vi "Rx Streaming (Host).vi"() -> ()   [LabVIEW 2015]
doc: "This template is for the Simple NI-USRP Streaming design, a design that shows the basics of streaming data to and from an NI USRP-294x/295x device. Refer to the block diagram for more information about how to use this template."
uses:
  <vilib>/userdefined/Silver/nirio_resource_slv.ctl
  SubVIs/Start Trigger.ctl
  <vilib>/Utility/error.llb/DialogType.ctl
  <vilib>/imath/engines/lvmath/Plug In/_Char/NIMS_CH_character datatype.ctl
  <instrlib>/niUsrpRio/Time/v1/Host/Private/Get Time (Single).vi
  Supporting Files/Global Vars.vi
  <vilib>/imath/engines/lvmath2/RunTimeEngine/Managers/WorkSpace/UID Generator.vi
  <vilib>/imath/engines/lvmath2/RunTimeEngine/BuiltInFunctions/close/NIMS_close(Enums).vi
  <vilib>/imath/engines/lvmath2/RunTimeEngine/RunTimeType/NIMS_RunTimeType_From StrictType (excl LVString).vi
  <instcachedir>/0/NIMS_RunTimeType_From StrictType (excl LVString)_EB1C38A9BC5048DA9ABDA8F781E54D21.lvgen/NIMS_RunTimeType_From StrictType (excl LVString)_EB1C38A9BC5048DA9ABDA8F781E54D21_000.vi
  <vilib>/imath/engines/lvmath2/RunTimeEngine/LocalVariableDefStatement/MC_LocalVariableDefStatement_Display.vi
  <vilib>/imath/engines/lvmath2/RunTimeEngine/BuiltInFunctions/log2/NIMS_log2(1o).vi
  <instcachedir>/0/NIMS_log2(1o)_7A1FF839A5EC4375BBB20124C6B1C03A.lvgen/NIMS_log2(1o)_7A1FF839A5EC4375BBB20124C6B1C03A_001.vi
  <vilib>/imath/engines/lvmath2/RunTimeEngine/RangeToken/NIMS_Range_R2 - Float.vi
  <instcachedir>/0/NIMS_Range_R2 - Float_98052C3F8D284261A146188355820AF0.lvgen/NIMS_Range_R2 - Float_98052C3F8D284261A146188355820AF0_000.vi
  <vilib>/imath/engines/lvmath2/RunTimeEngine/CommandStatement/MC_CommandStatement_break.vi
  <vilib>/imath/engines/lvmath2/RunTimeEngine/VariableToken/NIMS_VariableToken_CondDefined.vi
  <instcachedir>/0/NIMS_VariableToken_CondDefined_FE30D0A1BFB24F098D41DEBABFE96BE1.lvgen/NIMS_VariableToken_CondDefined_FE30D0A1BFB24F098D41DEBABFE96BE1_003.vi
  <vilib>/imathl/engines/lvmath/Functions/Error Handling/Create Error.vi
  <vilib>/imath/engines/lvmath2/RunTimeEngine/BuiltInFunctions/zeros/NIMS_V=zeros(I32,I32).vi
  <vilib>/imath/engines/lvmath2/RunTimeEngine/IndexRead/NIMS V(R2).vi
  <instcachedir>/0/NIMS V(R2)_C76619605A0E4E9F8B2FA9389712AC47.lvgen/NIMS V(R2)_C76619605A0E4E9F8B2FA9389712AC47_002.vi
  <vilib>/imath/engines/lvmath2/RunTimeEngine/ErrorHandling/NIMS_Create Error From Enums.vi
  <vilib>/imath/engines/lvmath2/RunTimeEngine/BuiltInFunctions/fftshift/NIMS_fftshift(GV).vi
  <instcachedir>/0/NIMS_fftshift(GV)_BD7A7BA9CA6B470B9A9F73A6A3FEEB3E.lvgen/NIMS_fftshift(GV)_BD7A7BA9CA6B470B9A9F73A6A3FEEB3E_000.vi
  <vilib>/imath/engines/lvmath2/RunTimeEngine/BuiltInFunctions/length/NIMS_length(GV).vi
  <instcachedir>/0/NIMS_length(GV)_08A3D13377FD4E4B96F5795FBF3698FA.lvgen/NIMS_length(GV)_08A3D13377FD4E4B96F5795FBF3698FA_004.vi
  <instcachedir>/0/NIMS V(R2)_C76619605A0E4E9F8B2FA9389712AC47.lvgen/NIMS V(R2)_C76619605A0E4E9F8B2FA9389712AC47_004.vi
  <vilib>/imath/engines/lvmath2/RunTimeEngine/BuiltInFunctions/fft/NIMS_fft(GV).vi
  <instcachedir>/0/NIMS_fft(GV)_4C6467FC22F84E4BA42517A07EF978B0.lvgen/NIMS_fft(GV)_4C6467FC22F84E4BA42517A07EF978B0_001.vi
  <instcachedir>/0/NIMS_fftshift(GV)_BD7A7BA9CA6B470B9A9F73A6A3FEEB3E.lvgen/NIMS_fftshift(GV)_BD7A7BA9CA6B470B9A9F73A6A3FEEB3E_001.vi
  <vilib>/imath/engines/lvmath2/RunTimeEngine/ErrorHandling/NIMS_Error From Error Code.vi
  <vilib>/imath/engines/lvmath2/RunTimeEngine/BuiltInFunctions/mean/NIMS_CS=mean(CV,I32).vi
  <vilib>/imath/engines/lvmath2/RunTimeEngine/RangeToken/NIMS_Range.vi
  <instcachedir>/0/NIMS_Range_D919CC09935940E88F755EC1C6F49AC1.lvgen/NIMS_Range_D919CC09935940E88F755EC1C6F49AC1_000.vi
  <vilib>/imath/engines/lvmath2/RunTimeSupport/NIMS_Error if Not Equal.vi
  <instcachedir>/0/NIMS_Error if Not Equal_7F0D61CE56BF44979916ECA34C78675F.lvgen/NIMS_Error if Not Equal_7F0D61CE56BF44979916ECA34C78675F_001.vi
  <vilib>/imath/engines/lvmath2/RunTimeEngine/IndexRead/NIMS V(V).vi
  <instcachedir>/0/NIMS V(V)_298D9CB7BFEB42B8BC8D9C3C28AE8C70.lvgen/NIMS V(V)_298D9CB7BFEB42B8BC8D9C3C28AE8C70_000.vi
  <vilib>/imath/engines/lvmath2/RunTimeEngine/ArithmeticOperatorToken/NIMS_ArithmeticOperator_times.vi
  <instcachedir>/0/NIMS_ArithmeticOperator_times_DF26C4080E2A467BA28C929B8CF31953.lvgen/NIMS_ArithmeticOperator_times_DF26C4080E2A467BA28C929B8CF31953_003.vi
  <vilib>/imath/engines/lvmath2/RunTimeEngine/BuiltInFunctions/sum/NIMS_sum(GV).vi
  <instcachedir>/0/NIMS_sum(GV)_67F5EC36BC034E54A6BEC5B0673C00E5.lvgen/NIMS_sum(GV)_67F5EC36BC034E54A6BEC5B0673C00E5_001.vi
  <vilib>/imath/engines/lvmath2/RunTimeEngine/BuiltInFunctions/conjugate/NIMS_conjugate(Complex).vi
  <instcachedir>/0/NIMS_conjugate(Complex)_151E186CA54B4853A0120BB0A667D86E.lvgen/NIMS_conjugate(Complex)_151E186CA54B4853A0120BB0A667D86E_001.vi
  <vilib>/imath/engines/lvmath2/RunTimeEngine/IndexRead/NIMS V(R3).vi
  <instcachedir>/0/NIMS V(R3)_BB7B7B2F47B844E7B6C44853B6A6C035.lvgen/NIMS V(R3)_BB7B7B2F47B844E7B6C44853B6A6C035_000.vi
  <instcachedir>/0/NIMS V(R2)_C76619605A0E4E9F8B2FA9389712AC47.lvgen/NIMS V(R2)_C76619605A0E4E9F8B2FA9389712AC47_001.vi
  <instcachedir>/0/NIMS_conjugate(Complex)_151E186CA54B4853A0120BB0A667D86E.lvgen/NIMS_conjugate(Complex)_151E186CA54B4853A0120BB0A667D86E_002.vi
  <vilib>/imath/engines/lvmath2/RunTimeEngine/ArithmeticOperatorToken/NIMS_ArithmeticOperator_minus.vi
  <instcachedir>/0/NIMS_ArithmeticOperator_minus_8228ED1EA52B4CB8A68367813E4B0C9D.lvgen/NIMS_ArithmeticOperator_minus_8228ED1EA52B4CB8A68367813E4B0C9D_000.vi
  <vilib>/imath/engines/lvmath2/RunTimeEngine/IndexReplace/NIMS V(R2)=V.vi
  <instcachedir>/0/NIMS V(R2)=V_A4A1DC5DDA874862BD08E3229D1DC268.lvgen/NIMS V(R2)=V_A4A1DC5DDA874862BD08E3229D1DC268_000.vi
  <vilib>/imath/engines/lvmath2/RunTimeEngine/BuiltInFunctions/ifft/NIMS_ifft(CV).vi
  <vilib>/imath/engines/lvmath2/RunTimeEngine/BuiltInFunctions/circularshift/NIMS_circularshift(GRowV,V).vi
  <instcachedir>/0/NIMS_circularshift(GRowV,V)_5CE594553FE04FE4B0327743CF19F361.lvgen/NIMS_circularshift(GRowV,V)_5CE594553FE04FE4B0327743CF19F361_000.vi
  <vilib>/imath/engines/lvmath2/RunTimeEngine/ArithmeticOperatorToken/NIMS_ArithmeticOperator_multmx(RV,CV).vi
  <instcachedir>/0/NIMS_ArithmeticOperator_multmx(RV,CV)_F97A2E11DB934918B28B7061ACE95B4F.lvgen/NIMS_ArithmeticOperator_multmx(RV,CV)_F97A2E11DB934918B28B7061ACE95B4F_000.vi
  <vilib>/imath/engines/lvmath2/RunTimeEngine/BuiltInFunctions/angle/NIMS_angle.vi
  <instcachedir>/0/NIMS_angle_6DDAE2BD99E0421EB990B6436E94D88F.lvgen/NIMS_angle_6DDAE2BD99E0421EB990B6436E94D88F_001.vi
  <instcachedir>/0/NIMS_Range_D919CC09935940E88F755EC1C6F49AC1.lvgen/NIMS_Range_D919CC09935940E88F755EC1C6F49AC1_001.vi
  <instcachedir>/0/NIMS_ArithmeticOperator_times_DF26C4080E2A467BA28C929B8CF31953.lvgen/NIMS_ArithmeticOperator_times_DF26C4080E2A467BA28C929B8CF31953_008.vi
  <instcachedir>/0/NIMS_ArithmeticOperator_times_DF26C4080E2A467BA28C929B8CF31953.lvgen/NIMS_ArithmeticOperator_times_DF26C4080E2A467BA28C929B8CF31953_001.vi
  <vilib>/imath/engines/lvmath2/RunTimeEngine/BuiltInFunctions/fft/NIMS_fft(GM).vi
  <instcachedir>/0/NIMS_fft(GM)_794D5E2C5B554C1782206BCB6828905B.lvgen/NIMS_fft(GM)_794D5E2C5B554C1782206BCB6828905B_001.vi
  <vilib>/imath/engines/lvmath2/RunTimeEngine/BuiltInFunctions/reshapemx/NIMS_[GM]_reshapemx(2i).vi
  <instcachedir>/0/NIMS_[GM]_reshapemx(2i)_50386BD9852D412C980AE89C68C2097F.lvgen/NIMS_[GM]_reshapemx(2i)_50386BD9852D412C980AE89C68C2097F_003.vi
  <vilib>/imath/engines/lvmath2/RunTimeEngine/BuiltInFunctions/sum/NIMS_sum(GM,Sca).vi
  <instcachedir>/0/NIMS_sum(GM,Sca)_AA1FD0B14F5C48868C267708D9376B4F.lvgen/NIMS_sum(GM,Sca)_AA1FD0B14F5C48868C267708D9376B4F_000.vi
  <vilib>/imath/engines/lvmath2/RunTimeEngine/IndexRead/NIMS V(S).vi
  <instcachedir>/0/NIMS V(S)_0488751826AF41519A22953C041130DC.lvgen/NIMS V(S)_0488751826AF41519A22953C041130DC_003.vi
  <vilib>/imath/engines/lvmath2/RunTimeEngine/IndexReplace/NIMS V(S)=S.vi
  <instcachedir>/0/NIMS V(S)=S_9916D32195284AEB9D40BA9A64F3B0C5.lvgen/NIMS V(S)=S_9916D32195284AEB9D40BA9A64F3B0C5_001.vi
  <vilib>/imath/engines/lvmath2/RunTimeEngine/BuiltInFunctions/conjugate/NIMS_conjugate(Real).vi
  <instcachedir>/0/NIMS_conjugate(Real)_2501B8F07B054B43A29FC6AFFF3C4398.lvgen/NIMS_conjugate(Real)_2501B8F07B054B43A29FC6AFFF3C4398_001.vi
  <instcachedir>/0/NIMS_ArithmeticOperator_times_DF26C4080E2A467BA28C929B8CF31953.lvgen/NIMS_ArithmeticOperator_times_DF26C4080E2A467BA28C929B8CF31953_009.vi
  <vilib>/imath/engines/lvmath2/RunTimeEngine/ArithmeticOperatorToken/NIMS_ArithmeticOperator_plus.vi
  <instcachedir>/0/NIMS_ArithmeticOperator_plus_A4F2756F5ADB4A0090E0DBD7C10701C8.lvgen/NIMS_ArithmeticOperator_plus_A4F2756F5ADB4A0090E0DBD7C10701C8_002.vi
  <instcachedir>/0/NIMS_ArithmeticOperator_minus_8228ED1EA52B4CB8A68367813E4B0C9D.lvgen/NIMS_ArithmeticOperator_minus_8228ED1EA52B4CB8A68367813E4B0C9D_008.vi
  <vilib>/imath/engines/lvmath2/RunTimeEngine/BuiltInFunctions/abs/NIMS_abs(signed).vi
  <instcachedir>/0/NIMS_abs(signed)_C4FCB8E6058B49B797C7C8D53CA5F6EC.lvgen/NIMS_abs(signed)_C4FCB8E6058B49B797C7C8D53CA5F6EC_003.vi
  <vilib>/imath/engines/lvmath2/RunTimeEngine/ArithmeticOperatorToken/NIMS_ArithmeticOperator_rightdivmx(C,C).vi
  <instcachedir>/0/NIMS_ArithmeticOperator_rightdivmx(C,C)_8AB7F1F477EE4166BF59ADE0F95BCF66.lvgen/NIMS_ArithmeticOperator_rightdivmx(C,C)_8AB7F1F477EE4166BF59ADE0F95BCF66_000.vi
  <vilib>/imath/engines/lvmath2/RunTimeEngine/BuiltInFunctions/max/2 inputs/NIMS_max(CA,CA).vi
  <instcachedir>/0/NIMS_max(CA,CA)_FEEF8ED63D764E06BBF554C779C98AAC.lvgen/NIMS_max(CA,CA)_FEEF8ED63D764E06BBF554C779C98AAC_000.vi
  <instcachedir>/0/NIMS_abs(signed)_C4FCB8E6058B49B797C7C8D53CA5F6EC.lvgen/NIMS_abs(signed)_C4FCB8E6058B49B797C7C8D53CA5F6EC_006.vi
  <vilib>/imath/engines/lvmath2/RunTimeEngine/RelationalOperatorToken/NIMS_Relational_Operator_Lt.vi
  <instcachedir>/0/NIMS_Relational_Operator_Lt_2B6DDA030731432BB98519CF5D23C4FD.lvgen/NIMS_Relational_Operator_Lt_2B6DDA030731432BB98519CF5D23C4FD_003.vi
  <vilib>/imath/engines/lvmath2/RunTimeEngine/BuiltInFunctions/findnz/NIMS_[1o]_findnz(GM).vi
  <instcachedir>/0/NIMS_[1o]_findnz(GM)_FAA59DEDB8D0486B8A0D06043103ACA4.lvgen/NIMS_[1o]_findnz(GM)_FAA59DEDB8D0486B8A0D06043103ACA4_003.vi
  <vilib>/imath/engines/lvmath2/RunTimeEngine/IndexReplace/NIMS V(M)=S.vi
  <instcachedir>/0/NIMS V(M)=S_EC01EE3B14AE4D46B4A839F4A346284F.lvgen/NIMS V(M)=S_EC01EE3B14AE4D46B4A839F4A346284F_000.vi
  <vilib>/imath/engines/lvmath2/RunTimeEngine/RangeToken/NIMS_Range_R2 - Integer.vi
  <instcachedir>/0/NIMS_Range_R2 - Integer_396D5D4FB869421F9245109A0975AD54.lvgen/NIMS_Range_R2 - Integer_396D5D4FB869421F9245109A0975AD54_000.vi
  <instcachedir>/0/NIMS_length(GV)_08A3D13377FD4E4B96F5795FBF3698FA.lvgen/NIMS_length(GV)_08A3D13377FD4E4B96F5795FBF3698FA_001.vi
  <instcachedir>/0/NIMS_abs(signed)_C4FCB8E6058B49B797C7C8D53CA5F6EC.lvgen/NIMS_abs(signed)_C4FCB8E6058B49B797C7C8D53CA5F6EC_002.vi
  <vilib>/imath/engines/lvmath2/RunTimeEngine/VariableToken/NIMS_VariableToken_CondDefinedDefinedByReplace.vi
  <instcachedir>/0/NIMS_VariableToken_CondDefinedDefinedByReplace_D162CFFC24174562A9FEA619A91E1A56.lvgen/NIMS_VariableToken_CondDefinedDefinedByReplace_D162CFFC24174562A9FEA619A91E1A56_000.vi
  <instcachedir>/0/NIMS_VariableToken_CondDefined_FE30D0A1BFB24F098D41DEBABFE96BE1.lvgen/NIMS_VariableToken_CondDefined_FE30D0A1BFB24F098D41DEBABFE96BE1_000.vi
  <vilib>/imath/engines/lvmath2/RunTimeEngine/BuiltInFunctions/min/1 input/NIMS_min(CV).vi
  <instcachedir>/0/NIMS_min(CV)_8813E20CADE24593A7CF0EDCC635D638.lvgen/NIMS_min(CV)_8813E20CADE24593A7CF0EDCC635D638_000.vi
  <vilib>/imath/engines/lvmath2/RunTimeEngine/BuiltInFunctions/figure/NIMS_figure(I32).vi
  <vilib>/imath/engines/lvmath2/RunTimeEngine/BuiltInFunctions/subplot/NIMS_subplot(I32, I32, I32).vi
  <vilib>/imath/engines/lvmath2/RunTimeEngine/BuiltInFunctions/plot/NIMS_plot(RM, RM, Str).vi
  <vilib>/imath/engines/lvmath2/RunTimeEngine/BuiltInFunctions/num_to_str/NIMS_num_to_str(GM,I32).vi
  <instcachedir>/0/NIMS_num_to_str(GM,I32)_5A43A194320A443797C56C876C2FDAAF.lvgen/NIMS_num_to_str(GM,I32)_5A43A194320A443797C56C876C2FDAAF_001.vi
  <vilib>/imath/engines/lvmath/Plug In/_Char/NIMS_CH_String CV to Character 2D.vi
  <instcachedir>/0/NIMS_CH_String CV to Character 2D_EC8CCB3F0D074D66A728E5B1D55F815A.lvgen/NIMS_CH_String CV to Character 2D_EC8CCB3F0D074D66A728E5B1D55F815A_000.vi
  <vilib>/imath/engines/lvmath2/RunTimeEngine/RowToken/NIMS_RowToken_SorRV_M.vi
  <instcachedir>/0/NIMS_RowToken_SorRV_M_3B0C3F1CE69D4FE0B3CF456C0E38D516.lvgen/NIMS_RowToken_SorRV_M_3B0C3F1CE69D4FE0B3CF456C0E38D516_001.vi
  <vilib>/imath/engines/lvmath/Plug In/_Char/NIMS_CH_Character RV to String.vi
  <vilib>/imath/engines/lvmath2/RunTimeEngine/BuiltInFunctions/title/NIMS_title.vi
  <vilib>/imath/engines/lvmath2/RunTimeEngine/BuiltInFunctions/ylabel/NIMS_ylabel.vi
  <vilib>/imath/engines/lvmath2/RunTimeEngine/BuiltInFunctions/xlabel/NIMS_xlabel.vi
  <vilib>/imath/engines/lvmath2/RunTimeEngine/BuiltInFunctions/axis/NIMS_axis.vi
  <vilib>/imath/engines/lvmath2/RunTimeEngine/BuiltInFunctions/grid/NIMS_grid.vi
  <vilib>/imath/engines/lvmath2/RunTimeEngine/BuiltInFunctions/max/1 input/NIMS_max(RV).vi
  <instcachedir>/0/NIMS_max(RV)_237633DB1D604D5BA7001287DF3C7957.lvgen/NIMS_max(RV)_237633DB1D604D5BA7001287DF3C7957_000.vi
  <vilib>/imath/engines/lvmath2/RunTimeEngine/BuiltInFunctions/hold/NIMS_hold(Enums).vi
  <vilib>/imath/engines/lvmath2/RunTimeEngine/RowToken/NIMS_RowToken_M_M.vi
  <instcachedir>/0/NIMS_RowToken_M_M_4D065800700C47988D760C22D4E255DD.lvgen/NIMS_RowToken_M_M_4D065800700C47988D760C22D4E255DD_003.vi
  <vilib>/imath/engines/lvmath2/RunTimeEngine/BuiltInFunctions/max/1 input/NIMS_max(CV).vi
  <instcachedir>/0/NIMS_max(CV)_A85366AFBDD24459900A7FDE15250013.lvgen/NIMS_max(CV)_A85366AFBDD24459900A7FDE15250013_000.vi
  <vilib>/imath/engines/lvmath2/RunTimeEngine/BuiltInFunctions/num_to_str/NIMS_num_to_str(GRowV,I32).vi
  <instcachedir>/0/NIMS_num_to_str(GRowV,I32)_8449A5A7B42346CF9378CDDB5FBEA53D.lvgen/NIMS_num_to_str(GRowV,I32)_8449A5A7B42346CF9378CDDB5FBEA53D_001.vi
  <vilib>/imath/engines/lvmath/Plug In/_Char/NIMS_CH_String to Character Array.vi
  <vilib>/imath/engines/lvmath2/RunTimeEngine/Managers/SymbolTable/Clear UID.vi
  <vilib>/imath/engines/lvmath2/RunTimeEngine/ErrorHandling/NIMS_Finalize Error.vi
  <instrlib>/niUsrpRio/Time/v1/Host/niUsrpRio Time v1 Host.lvlib
  <instrlib>/niUsrpRio/Config/v1/Host/niUsrpRio Config v1 Host.lvlib
  <vilib>/imath/engines/lvmath2/RunTimeEngine/Managers/SymbolTable/NIMS_WorkSpace.lvlib
panel:
  out "Boolean":bool
  out "GPS Lock Time Elapsed":dbl format="%<%H:%M:%S>t"
  in  "Frequency\nauto-correction":bool
  in  "Display graphs":bool
  out "Matlab Error":errorcluster
  out "Block no.":i32
  in  "No. of blocks \nto receive":i32=5
  out "Debugging data":csg[](array[numeric])
  in  "Read file from hardisk for debugging":path=path "C:/Users/ctme/Documents/Test Data/Recieved_Data"
  in  "Rx data update \ninterval (seconds)":dbl=1.0 format="%#_13g"
  out "File write error":errorcluster
  in  "Write to HDD":path=path "C:/Users/ctme/Documents/Test Data/Recieved_Data"
  out "RX data IQ":cdb[](array[numeric])
  in  "config tab":enum32{"Rx Configuration"}(tab)
  in  "rx config":T2={"rf enable 0"=TRUE, "rf config 0"={"antenna"="RX2", "frequency"=5800000000.0, "lo frequency"=-1.0, "level"=30.0}, "rf enable 1"=FALSE, "rf config 1"={"antenna"="RX2", "frequency"=2000000000.0, "lo frequency"=-1.0, "level"=0.0}, "number of samples is finite"=TRUE, "sample rate"=200000000.0, "number of samples"=262160, "start trigger"=enum."Immediate"} {"sample rate" format="%#.3pS/s"; "rf config 1"."level" format="%#_gdB"; "rf config 1"."lo frequency" format="%#.3pHz"; "rf config 1"."frequency" format="%#.3pHz"; "rf config 0"."level" format="%#_gdB"; "rf config 0"."lo frequency" format="%#.3pHz"; "rf config 0"."frequency" format="%#.3pHz"}
  out "acquiring":bool caption="Acquiring"
  in  "USRP RIO device":T3="RIO0" caption="USRP RIO Device"
  in  "reference frequency source":string(combo)="Internal" caption="Reference Frequency Source"
  in  "indicator tab":T4(tab)
  out "power spectrum":cluster{"f0":dbl, "df":dbl, "magnitude":dbl[]}[](graph) caption="Power Spectrum"
  out "power level":dbl[][](graph) caption="Power Level"
  out "iq data":dbl[][](graph) caption="I & Q Data"
  out "rx.coerced config":T5 caption="Rx" {"coerced sample rates" format="%#.3pS/s"; "coerced levels" format="%#.3gdB"; "coerced lo frequencies" format="%#.3pHz"; "coerced frequencies" format="%#.3pHz"}
  in  "rx.stop":bool
  # "Victoria University - Telstra \n5G mm-wave measurement - Receiver"
  # "Simple Rx Streaming"
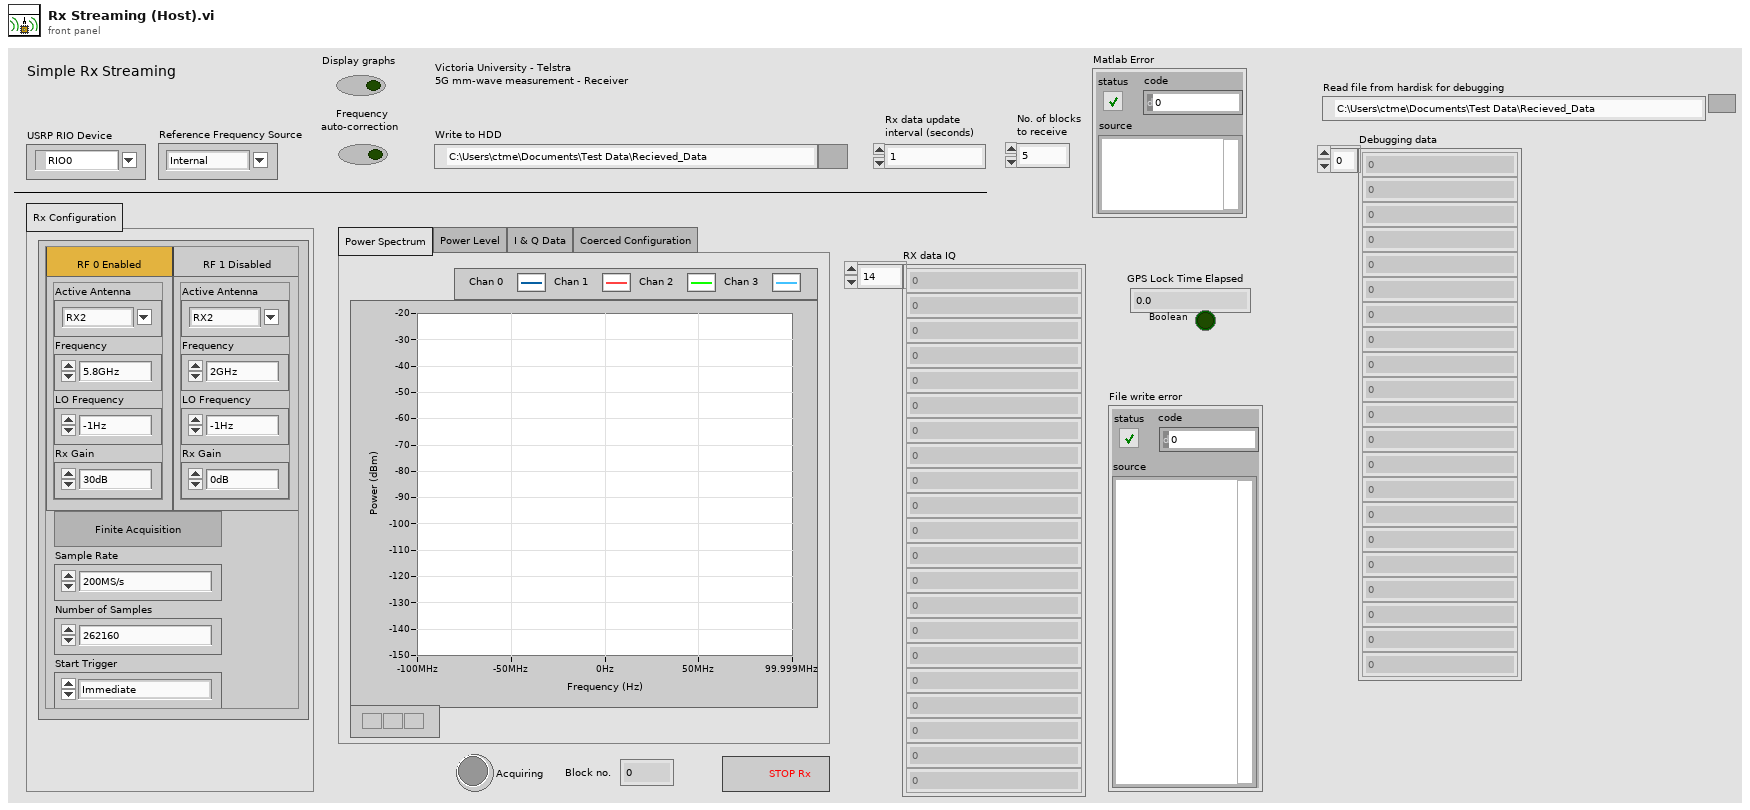
[diagram p1: front panel]
types:
  T1 = typedef "Start Trigger.ctl" = enum8{"Software", "Digital Edge", "Rx Start Trigger", "Tx Start Trigger", "Immediate", "Future Time Event"}
  T2 = cluster{"rf enable 0":bool, "rf config 0":cluster{"antenna":string, "frequency":dbl, "lo frequency":dbl, "level":dbl}, "rf enable 1":bool, "rf config 1":cluster{"antenna":string, "frequency":dbl, "lo frequency":dbl, "level":dbl}, "number of samples is finite":bool, "sample rate":dbl, "number of samples":u32, "start trigger":T1}
  T3 = typedef "nirio_resource_slv.ctl" = tag
  T4 = enum32{"Power Spectrum", "Power Level", "I & Q Data", "Coerced Configuration"}
  T5 = cluster{"coerced frequencies":dbl[], "coerced lo frequencies":dbl[], "coerced levels":dbl[], "coerced sample rates":dbl[]}
  T6 = typedef "DialogType.ctl" = u16
  T7 = enum16{"open", "replace", "create", "open or create", "replace or create", "replace or create with confirmation"}
  T8 = cluster{"rx config":cluster{"rf enable 0":bool, "rf config 0":cluster{"antenna":string, "frequency":dbl, "lo frequency":dbl, "level":dbl}, "rf enable 1":bool, "rf config 1":cluster{"antenna":string, "frequency":dbl, "lo frequency":dbl, "level":dbl}, "number of samples is finite":bool, "sample rate":dbl, "number of samples":u32, "start trigger":T1}, "reference frequency source":string, "rx.enabled channels":string[], "vertical range":dbl[], "rx.coerced configurations":cluster{"coerced frequencies":dbl[], "coerced lo frequencies":dbl[], "coerced levels":dbl[], "coerced sample rates":dbl[]}}
  T9 = typedef "niUsrpRio Config v1 Host.lvlib/niUsrpRio Session.ctl" = cluster{"FPGA Interface":refnum<k20>, "RIO Interface Number":u32, "Data Clock Rate":u32, "FPGA Data Clock Rate":u32, "Global Settings Register Bus":T10, "Radio 0 Settings Register Bus":T10, "Radio 1 Settings Register Bus":T10, "Radio Settings Bus Semaphore":T11, "DB Queues":T12[], "Characterization Data Valid?":bool, "EEPROM Header":T13, "Device Data Header":T14, "EEPROM Characterization Header":T15, "Characterization Data":T16[], "FPGA Current Version":u32, "FPGA Oldest Compatible Version":u32, "Fixed Logic Current Version":u32, "Fixed Logic Oldest Compatible Version":u32, "FPGA Radio Settings Bus Current Version":u32, "FPGA Radio Settings Bus Oldest Compatible Version":u32, "FPGA Board Config Current Version":u32, "FPGA Board Config Oldest Compatible Version":u32}
  T10 = typedef "niInstr Register Bus v0 Host.lvlib/Register Bus Session.ctl" = refnum<queue>
  T11 = typedef "Semaphore RefNum" = refnum<k1>
  T12 = typedef "niUsrpRio Config v1 Host.lvlib/DB Queue Reference.ctl" = refnum<queue>
  T13 = typedef "niUsrpRio Config v1 Host.lvlib/EEPROM Header.ctl" = cluster{"Checksum":u32, "Product Code":u16, "Hardware Current Version":u16, "Hardware Oldest Compatible Version":u16, "EEPROM Map Current Version":u16, "EEPROM Map Oldest Compatible Version":u16, "User Password":string, "Pointer to Factory Header":u32, "Pointer to User Header":u32, "Recommended Interval":u16, "Number of Reserved Bytes":i32, "Number of Daughterboards":u8, "Daughterboard IDs":u16[], "Daughterboard Serial Numbers":string[]}
  T14 = typedef "niUsrpRio Config v1 Host.lvlib/EEPROM Device Data Header.ctl" = cluster{"Checksum":u32, "Number of Channels":u8, "Number of Gain Settings":u16[], "Pointer to Characterization Data":u32[], "Number of Reserved Bytes":i32, "Number of Frequencies":u16[]}
  T15 = typedef "niUsrpRio Config v1 Host.lvlib/EEPROM Characterization Header.ctl" = cluster{"Checksum":u32, "Date":timestamp, "Temperature":sgl, "Misc. Info":string, "Pointer to Device Data Header":u32, "Number of Reserved Bytes":i32}
  T16 = typedef "niUsrpRio Config v1 Host.lvlib/Characterization Data.ctl" = cluster{"Gains[dB]":dbl[], "Frequencies [Hz]":dbl[], "IQ Imbalance Table":T17[], "Measured Gains[dB]":dbl[][]}
  T17 = typedef "niUsrpRio Config v1 Host.lvlib/IQ Imbalance.ctl" = cluster{"Gain Imbalance [linear]":dbl, "Phase Imbalance [radians]":dbl, "Offset":cdb}
  T18 = enum16{"big-endian, network order", "native, host order", "little-endian"}
  T19 = typedef "NIMS_CH_character datatype.ctl" = cluster{"Numeric":u8}
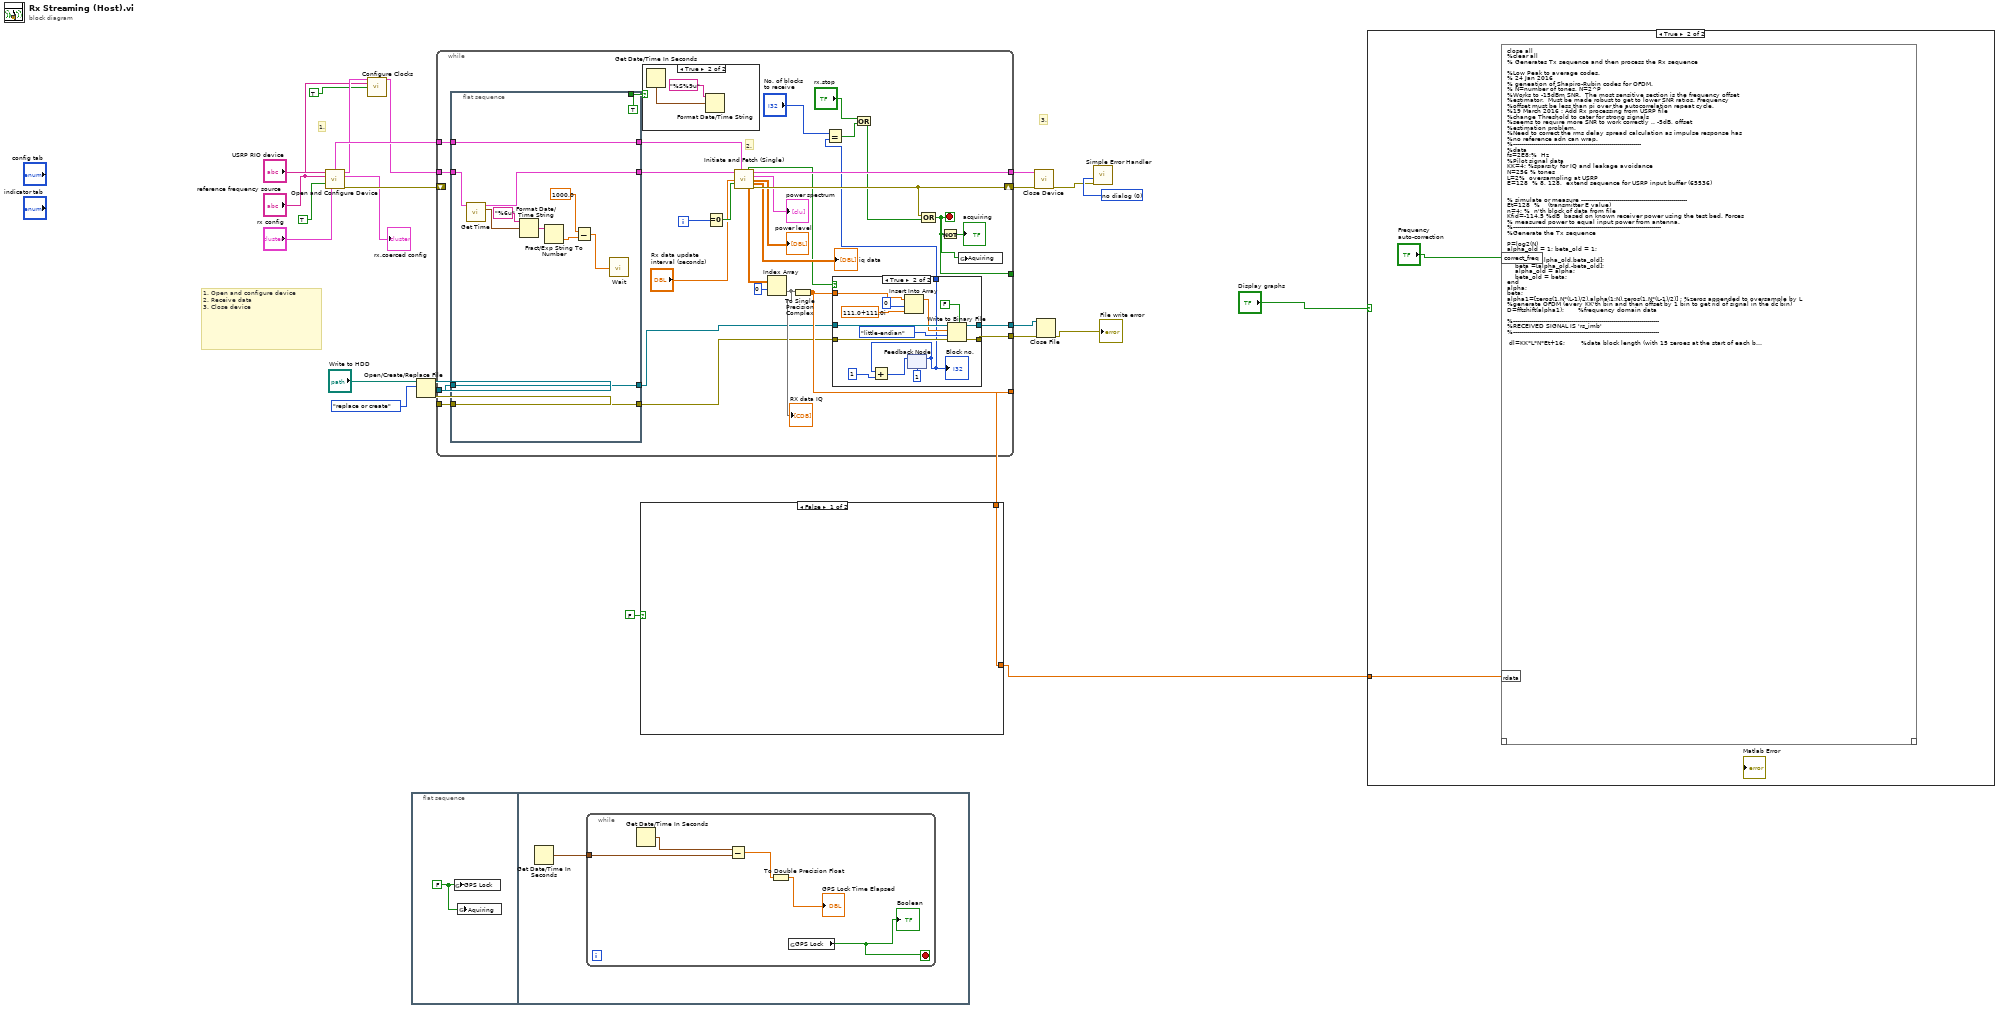
[diagram p0: block diagram]
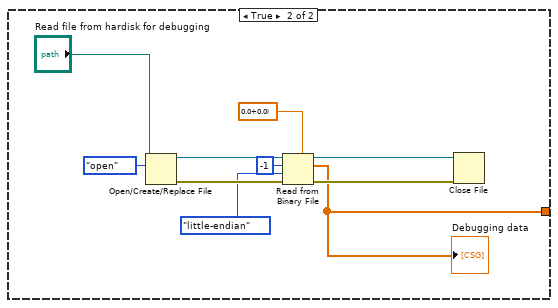
[diagram p3: hidden frame]
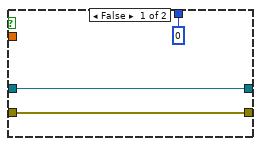
[diagram p5: hidden frame]
diagram:
  w11 = T6 0 items=["no dialog", "OK message", "continue or stop message", "OK message + warnings", "continue/stop + warnings"] ("type of dialog (OK msg:1)")
  # "3."
  # "1. Open and configure device\n2. Receive data\n3. Close device"
  # "1."
  n1 = call "Open and Configure Device.vi"("USRP RIO Device"="USRP RIO device", "reference frequency source"="reference frequency source", "Wait for GPS Lock?"=TRUE, "rx config"="rx config") -> ("rx channels"=w24:T8, "niUsrpRio Session (out)"=w6:T9, "rx.coerced configurations"=→"rx.coerced config":T5, "error out"=w25:errorcluster)  [unwired: 6 in, 2 out]
  n2 = call <instrlib>:"Configure Clocks.vi"("niUsrpRio Session"=w6, "Reference Frequency Source"="reference frequency source", "GPSDO Power Enable"=TRUE) -> ("niUsrpRio Session (out)"=w5:T9)  [unwired: 11 in, 1 out]
  n3 = flat-sequence {
    frame #0 {
      w26 = FALSE
      n4 = global write "Global Vars.vi" "GPS Lock"(w26) -> ()
      n5 = global write "Global Vars.vi" "Aquiring"(w26) -> ()
    }
    frame #1 {
      n6 = Get Date/Time In Seconds() -> (seconds since 1Jan1904=w27:timestamp)
      n7 = while {
        tunnel: w27 -> [w30]
        stop <- w28 stop-if-true
        n8 = Get Date/Time In Seconds() -> (seconds since 1Jan1904=w29:timestamp)
        n9 = Subtract(x=w29, y=w30) -> (x-y=w32:dbl)
        n10 = To Double Precision Float(number=w32) -> (double precision float=→"GPS Lock Time Elapsed":dbl)
        n11 = global read "Global Vars.vi" "GPS Lock"() -> (w28:bool)
        "Boolean" <- w28
      }
    }
  }
  n12 = Open/Create/Replace File(file path (use dialog)="Write to HDD", operation (0:open)=T7."replace or create") -> (refnum out=w16:refnum<file>, error out=w15:errorcluster)  [unwired: 4 in, 1 out]
  n13 = while {
    tunnel: w5 -> [w37]
    tunnel: [w62] -> w20
    tunnel: w24 -> [w38]
    shift-right: [w63] -> w21
    shift-left: w25 -> [_]
    tunnel: w16 -> [w42]
    tunnel: w15 -> [w39]
    tunnel: [w54] -> w14
    tunnel: [w53] -> w13
    tunnel: [w33] -> _
    tunnel: [w50] -> w8
    i -> [w48]
    stop <- w33 stop-if-true
    # "2."
    # "Acquire and Fetch a waveform"
    n14 = flat-sequence {
      tunnel: [TRUE] -> w43
      tunnel: [w74] -> w41
      tunnel: w42 -> [w74]
      tunnel: [w73] -> w40
      tunnel: w39 -> [w73]
      tunnel: w38 -> [w72]
      tunnel: w37 -> [w71]
      tunnel: [w70] -> w36
      tunnel: [w72] -> w35
      frame #0 {
        n15 = call-poly <instrlib>:"Get Time.vi"("niUsrpRio Session"=w71) -> ("niUsrpRio Session (out)"=w70:T9, "time"=w69:timestamp)  [unwired: 12 in, 1 out]
        n16 = Format Date/Time String(time format string (%c)="%6u", seconds (now)=w69) -> (date/time string=w67:string)  [unwired: 1 in]
        n17 = Fract/Exp String To Number(string=w67) -> (number=w66:dbl)  [unwired: 3 in, 1 out]
        n18 = Subtract(x=1000.0, y=w66) -> (x-y=w65:dbl)
        n19 = call "Wait"("Count(uSec)"=w65) -> ()  [unwired: 1 out]
      }
    }
    n20 = case shown="True" w43 {
      frame False {
      }
      frame True {
        n21 = Get Date/Time In Seconds() -> (seconds since 1Jan1904=w77:timestamp)
        n22 = Format Date/Time String(time format string (%c)="%S%9u", seconds (now)=w77) -> ()  [unwired: 1 in, 1 out]
      }
    }
    n23 = Equal To 0?(x=w48) -> (x = 0?=w58:bool)
    n24 = call "Initiate and Fetch (Single).vi"("niUsrpRio Session"=w36, "rx channels"=w35, "update interval"="Rx data update \ninterval (seconds)", "first iteration"=w58) -> ("Time has Elapsed"=w52:bool, "niUsrpRio Session (out)"=w62:T9, "power spectrum"=→"power spectrum":cluster{"f0":dbl, "df":dbl, "magnitude":dbl[]}[], "power level"=→"power level":dbl[][], "iq data"=→"iq data":dbl[][], "complex baseband data"=w56:cdb[][], "error out"=w63:errorcluster)  [unwired: 5 in]
    n25 = Index Array(array=w56, index (row)=0) -> (element=w51:cdb[])  [unwired: 1 in]
    "RX data IQ" <- w51
    n26 = To Single Precision Complex(1:w51) -> (0:w50:csg[])
    n27 = case shown="True" w52 {
      tunnel: w41 -> [w80 w92]
      tunnel: w40 -> [w79 w91]
      tunnel: [w80 w90] -> w54
      tunnel: [w79 w89] -> w53
      tunnel: w50 -> [_ w86]
      tunnel: [0 w82] -> w45
      frame False {
      }
      frame True {
        n28 = Insert Into Array(array=w86, index=0, new element=csg 111.0+111.0i ("new element/subarray")) -> (w85:csg[])
        n29 = feedback #1(1) -> (w82:i32)
        "Block no." <- w82
        n30 = Add(x=w82, y=1) -> (x+y=w83:i32)
        n31 = feedback-in #1(w83) -> ()
        n32 = Write to Binary File(file (use dialog)=w92, data=w85, error in=w91, 5:FALSE ("prepend array or string size? (T)"), 9:T18."little-endian" ("byte order (0:big-endian, network order)")) -> (refnum out=w90:refnum<file>, error out=w89:errorcluster)  [unwired: 1 in, 1 out]
      }
    }
    n33 = Equal?(x="No. of blocks \nto receive", y=w45) -> (x = y?=w47:bool)
    n34 = Or(x="rx.stop", y=w47) -> (x .or. y?=w44:bool)
    n35 = Compound Arithmetic op=OR(w63, w44) -> (w33:bool)
    n36 = Not(x=w33) -> (.not. x?=→"acquiring":bool)
    n37 = global write "Global Vars.vi" "Aquiring"(w33) -> ()
  }
  n38 = case shown="False" FALSE {
    tunnel: [w95 w96] -> w1
    tunnel: w8 -> [w95 _]
    frame False {
    }
    frame True {
      n39 = Open/Create/Replace File(file path (use dialog)="Read file from hardisk for debugging", operation (0:open)=T7."open") -> (refnum out=w103:refnum<file>, error out=w101:errorcluster)  [unwired: 4 in, 1 out]
      n40 = Read from Binary File(5:csg 0.0+0.0i ("Array"), 8:w101, 9:T18."little-endian" ("byte order (0:big-endian, network order)"), 10:-1 ("count (1)"), 11:w103) -> (0:w100:errorcluster, 2:w96:csg[], 3:w102:refnum<file>)  [unwired: 1 in, 1 out]
      "Debugging data" <- w96
      n41 = Close File(refnum=w102, error in=w100) -> ()  [unwired: 2 out]
    }
  }
  n42 = call "Close Device.vi"("niUsrpRio Session"=w20, "error in"=w21) -> ("error out"=w10:errorcluster)  [unwired: 13 in]
  n43 = Close File(refnum=w14, error in=w13) -> (error out=→"File write error":errorcluster)  [unwired: 1 out]
  n44 = call <vilib>:"Simple Error Handler.vi"("type of dialog (OK msg:1)"=w11, "error in (no error)"=w10) -> ()  [unwired: 3 in, 5 out]
  n45 = case shown="True" "Display graphs" {
    tunnel: w1 -> [_ w106]
    frame False {
    }
    frame True {
      n46 = mathscript code="close all\n%clear all\n% Generates Tx sequence and then process the Rx sequence\n\n%Low Peak to average codes.\n% 24 Jan 2016\n% geneation of Shapiro-Rubin codes for OFDM. \n% N=number of tones, N=2^P\n%Works to -15dBm SNR.  The most sensitive section is the frequency offset\n%estimator.  Must be made robust to get to lower SNR ratios. Frequency\n%offset must be less than pi over the autocorrelation repeat cycle.\n%19 March 2016 : Add Rx processing from USRP file\n%change Threshold to cater for strong signals\n%seems to require more SNR to work correctly .. -5dB, offset\n%estimation problem.\n%Need to correct the rms delay spread calculation as impulse response has\n%no reference adn can wrap.\n%----------------------------------------------------------------\n%data\nfs=2E8;%  Hz\n%Pilot signal data\nKK=4; %sparsity for IQ and leakage avoidance \nN=256 % tones\nL=2%  oversampling at USRP\nE=128  % 8, 128,  extend sequence for USRP input buffer (65536)\n\n\n% simulate or measure -----------------------------------------------------\nEt=128  %    (transmitter E value)\nn=4; %  n'th block of data from file\nKfid=-114.5 %dB  based on known receiver power using the test bed. Forces \n% measured power to equal input power from antenna. \n%--------------------------------------------------------------------------\n%Generate the Tx sequence\n\nP=log2(N)\nalpha_old = 1; beta_old = 1;\nfor p = 1:P\n    alpha=[alpha_old,beta_old];\n    beta =[alpha_old,-beta_old];\n    alpha_old = alpha;\n    beta_old = beta;\nend\nalpha;\nbeta;\nalpha1=[zeros(1,N*(L-1)/2),alpha(1:N),zeros(1,N*(L-1)/2)] ; %zeros appended to oversample by L\n%generate OFDM (every KK'th bin and then offset by 1 bin to get rid of signal in the dc bin)\nD=fftshift(alpha1);       %frequency domain data\n\n%-------------------------------------------------------------------------\n%RECEIVED SIGNAL IS 'rs_imb'\n%-------------------------------------------------------------------------\n\n dl=KK*L*N*Et+16;        %data block length (with 15 zeroes at the start of each blk\n %rdata=read_complex_binary([filename],3*(dl+1)); %data blocks separated by a single \"1\" \nif (length(rdata)==262160)\nrs_block=rdata(16:end);%selecting the nth block (removing the 15 zeros and and block markers)\nelse\nrs_block=(rdata(n+(n-1)*dl+15+1:n+n*dl-1)); \nend\n rs_imb=rs_block(1:KK*L*N*E);\n RS_imb=fftshift(fft(rs_imb))/(KK*E); %used for plotting.   Scale to account for longer sequence \n \n%estimate Rx error first.  \n%The first bin contains DC if the averaging is much longer than 1/f_offset\ndc_rx_estimate=mean(rs_imb)\nrs_imb_mdc=rs_imb-dc_rx_estimate;        %remove dc offset\nRS_imb_mdc=fft(rs_imb_mdc);              %frequency domain\n\n%estimate image coefficient 'image_rx'\n%Close in quadrature errors are obtained by correlating image bins over\n%approx half the bandwidth\n%Correlate bins and divide by power (correct for power increase due to\n%image enhancement by iteration; one iteration is enough in most cases)\n%Here we use 4 iterations.  See Notes pg24.\n%Corr=RS_imb_mdc(2:N*KK*E/2)*(RS_imb_mdc(N*L*KK*E:-1:N*L*KK*E-N*KK*E/2+2).')\nCorrA=RS_imb_mdc(2:N*KK*E/2);\nCorrB=RS_imb_mdc(N*L*KK*E:-1:N*L*KK*E-N*KK*E/2+2);\nCorr=sum(CorrA.*CorrB)\n%Energy=RS_imb_mdc(2:N*KK*E/2)*RS_imb_mdc(2:N*KK*E/2)'+RS_imb_mdc(N*L*KK*E:-1:N*L*KK*E-N*KK*E/2+2)*RS_imb_mdc(N*L*KK*E:-1:N*L*KK*E-N*KK*E/2+2)'\nEnergyA1=RS_imb_mdc(2:N*KK*E/2);\nEnergyA2=conj(RS_imb_mdc(2:N*KK*E/2));\nEnergyB1=RS_imb_mdc(N*L*KK*E:-1:N*L*KK*E-N*KK*E/2+2);\nEnergyB2=conj(RS_imb_mdc(N*L*KK*E:-1:N*L*KK*E-N*KK*E/2+2));\nEnergy=sum(EnergyA1.*EnergyA2)+sum(EnergyB1.*EnergyB2);\n\nimage_rx_estimate=Corr/Energy %  first approximation\nimage_rx_estimate=(1+image_rx_estimate*image_rx_estimate')*Corr/Energy %2nd iteration\nimage_rx_estimate=(1+image_rx_estimate*image_rx_estimate')*Corr/Energy %3rd iteration\nimage_rx_estimate=(1+image_rx_estimate*image_rx_estimate')*Corr/Energy %4th iteration\n\n%correct for rx IQ imballance. Subtract image and correct gain\n%RS_correct = [0,RS_imb_mdc(2:N*L*KK*E) - image_rx_estimate .* conj(RS_imb_mdc(N*L*KK*E:-1:2))]/(1-image_rx_estimate*conj(image_rx_estimate));\nRS_correctA = [RS_imb_mdc(2:N*L*KK*E) - image_rx_estimate .* conj(RS_imb_mdc(N*L*KK*E:-1:2))]/(1-image_rx_estimate*conj(image_rx_estimate));\nRS_correct=zeros(1,N*L*KK*E);\nRS_correct(2:N*L*KK*E)=RS_correctA;\n\nif correct_freq\n    %% NOT REQUIRED FOR GPS LOCK\n    %use auto correlation to identify the freq offset\n    rs_correct=ifft(RS_correct);\n    rs_correct_delay = circshift(rs_correct,[0,N*L*KK]);\n    auto_cor=rs_correct(N*L*KK+1:end)*(rs_correct_delay(N*L*KK+1:end))';\n    f_offset_estimate=angle(auto_cor)/(N*L*KK);  %radians/sample\n\n    %correct frequency offset\n    rs_corrected_freqoffset= rs_correct.*exp(-1i.*f_offset_estimate.*[0:N*L*KK*E-1]);\n    RS_corrected_freqoffset=fft(rs_corrected_freqoffset);%check spectrum\nelse\n    %% REQUIRED FOR GPS LOCK--------------------------------------\n    rs_corrected_freqoffset=ifft(RS_correct);\nend\n\nclose all\n%clear all\n% Generates Tx sequence and then process the Rx sequence\n\n%Low Peak to average codes.\n% 24 Jan 2016\n% geneation of Shapiro-Rubin codes for OFDM. \n% N=number of tones, N=2^P\n%Works to -15dBm SNR.  The most sensitive section is the frequency offset\n%estimator.  Must be made robust to get to lower SNR ratios. Frequency\n%offset must be less than pi over the autocorrelation repeat cycle.\n%19 March 2016 : Add Rx processing from USRP file\n%change Threshold to cater for strong signals\n%remove repititions by avearaging the E repetitions of the signal\nrs=sum(reshape(rs_corrected_freqoffset,[N*L*KK,E]),2)/E;\nRS=fft(rs)/KK;  %spectrum (scale to line up with synthetic channel inputs, D)\ndc_tx_estimate=RS(1)\n%remove dc rotate back 1 bin, pick out the data bins, divide by the Txdata \n% obtain the delay spread \nRS(1)=0;\nRS_shift=circshift(RS.',[0,-1]);  %shift back\nR=RS_shift(1:KK:end) ;         % remove unused bins \nChannel = R.* conj(D);         % remove effect of input sequence to give channel\n\n%Estimate rx_SNR processing (before averaging) by measuring signal powers in the blank bins (frequency domain)\n%Noise_est=2*(RS_shift(2:KK/2:end))*(RS_shift(2:KK/2:end))' %blank bins\n%Signal_est=(RS_shift(1:KK:end))*(RS_shift(1:KK:end))' - Noise_est  %assumes noise per bin is the same\n%SNR_est=10*log10(Signal_est/Noise_est)\n\n%Estimate rx_SNR post-processing (after averaging) by measuring noise powers in the blank bins (frequency domain)\n%measureing signal powers in signal bins and subtract an estimate of the\n%noise component\nNoise_est=((RS_shift(2:KK/2:end/4))*(RS_shift(2:KK/2:end/4))'+(RS_shift(end:-KK/2:end-N*KK/2+1))*(RS_shift(end:-KK/2:end-N*KK/2+1))')/ (N*KK/2) %noise power per bin (averaged over blank bins)\nSignal_est=abs(((RS_shift(1:KK:N*KK/2))*(RS_shift(1:KK:N*KK/2))'+ (RS_shift(end-KK+1:-KK:end-N*KK/2))*(RS_shift(end-KK+1:-KK:end-N*KK/2))')/N  -  Noise_est) %signal power per bin = bin power -noise power/bin\nSNR_est=10*log10(abs(Signal_est/Noise_est))\n\nRxSignalPower=10*log10(Signal_est)+10*log10(N)+Kfid\n\n%---------------------------------------------------------------\n%channel processing\ncir_est=ifft(Channel);                      %impulse response\n\n%rms delay spread\n%calcuate threshold based on Noise_est. After correlation using the ifft \n%the noise per sample is furhter reduced by 1/N \n%Take the noise level and set the signal threshold power 10dB x\n%higher to minimise probability of peak going over threshold. Use 12dB if \n%required to be more cnservative \n%Note at strong signal levels, the delay spread is effected by the sinc\n%roll-off and low noise reduces the threshold and makes it worse! Works\n%best with SNRs of about 0dB!\n\nThreshold_n=sqrt(Noise_est*2.5/N)            %above the noise power. reduce from 10 to 2.5\nThreshold_s=sqrt(Signal_est/(8*N))          %below the signal power\nThreshold = max(Threshold_n,Threshold_s)    %highest\n\n%cir_h=wthresh(cir_est,'h',Threshold);\ncir_h=cir_est;\ncir_h(find(abs(cir_est)<Threshold))=0;\n% rotate impulse response until all components do not wrap (to give correct \n%lowest delay spread) \nfor shift=1:8 \n    cir_h=circshift(cir_h,[0,length(cir_h)/8]);\n    aat=0;aa=0;aatt=0;\n    for i=1:length(cir_h);   \n        aat=aat+i*(abs(cir_h(i))^2);\n        aa=aa+abs(cir_h(i))^2;\n        aatt=aatt+(i^2)*(abs(cir_h(i))^2);\n    end\nmse_delayspread = aatt/aa - (aat/aa)^2;\nrms_delayspread(shift) = sqrt(mse_delayspread);\nend\nrms_delay=min(rms_delayspread)\n\ncoherenceBW_50=1/(5*rms_delay)\ncoherenceBW_90=1/(50*rms_delay)\n\nfigure(1)\nsubplot(2,2,1)\nplot([-N*E*L*KK/2:1:N*E*L*KK/2-1]*fs/(N*E*L*KK),20*log10(abs(RS_imb)))\ntitle(['RX spectrum','; Signal pow= ',num2str(RxSignalPower),'dBm','; SNDR est= ',num2str(SNR_est-10*log10(E)),'dB' ]);ylabel(['dB']);xlabel(['frequency, Hz'])\naxis([-fs/2,(N*E*L*KK/2-1)*fs/(N*E*L*KK), -40,60]); grid\n\nsubplot(2,2,2)\n%plot((abs(Channel)))\nplot([-N*L/2:1:N*L/2-1]*fs/(L*N),fftshift(20*log10(abs(Channel)+0.01)))\ntitle(['Channel(f); SNRest=',num2str(SNR_est),'dB/bin'])\nylabel('dB'), grid\n\nsubplot(2,2,3)\nplot([0:N*L-1],abs(cir_est))\ntitle(['Threshold wrt strongest ray= ',num2str(20*log10(Threshold/max(abs(cir_est)))),'dB'])\nhold on\nplot([0,N*L-1],[Threshold,Threshold])\nhold off\nsubplot(2,2,4)\n[max_h, pos_hmax]=max(cir_h)          %put max impulse in the first 1/8\ncir_h=circshift(cir_h,[0,(length(cir_h)/8-pos_hmax)]); \nplot([-N*L/16:1:N*L*3/16-1]/fs,abs(cir_h(N*L/16:1:N*L*5/16-1)));\n%axis([(-N*L/16)/fs,(N*L*3/16-1)/fs,0,1])\ntitle(['Impulse Response','; RMS delay spread = ',num2str(rms_delay/fs), 's']); xlabel('seconds')\n\n%text(0.3,0.4,['Active tones=',num2str(N)])\n%,'string',['repititions, E=',num2str(E),', ==',num2str(10*log10(E)),'dB'])\n\n%Close in quadrature errors are obtained by correlating image bins over\n%approx half the bandwidth\n%image_estimate = RS_imb(2:KK*N*E/4)*RS_imb(KK*N*E:-1:2+KK*N*E*3/4)'"("rdata"=w106, "correct_freq"="Frequency\nauto-correction") -> ()  [unwired: 1 in, 1 out]
    }
  }
